vi "Write configuration.vi"(8 "error in":errorcluster, 10 "configuration":refnum<class "NISE_CEF_serializable configuration.lvclass">, 11 "My Awesome Control Modules editor node in":refnum<class "My Awesome Control Modules editor node.lvclass">) -> (0 "error out":errorcluster, 3 "My Awesome Control Modules editor node out":refnum<class "My Awesome Control Modules editor node.lvclass">)   [LabVIEW 2013, in "My Awesome Control Modules editor node.lvclass"]
uses:
  My Awesome Control Modules editor node.lvclass
  module/configuration/My Awesome Control Modules configuration.lvclass
  <vilib>/NI/Configuration Framework/serializable configuration/NISE_CEF_serializable configuration.lvclass
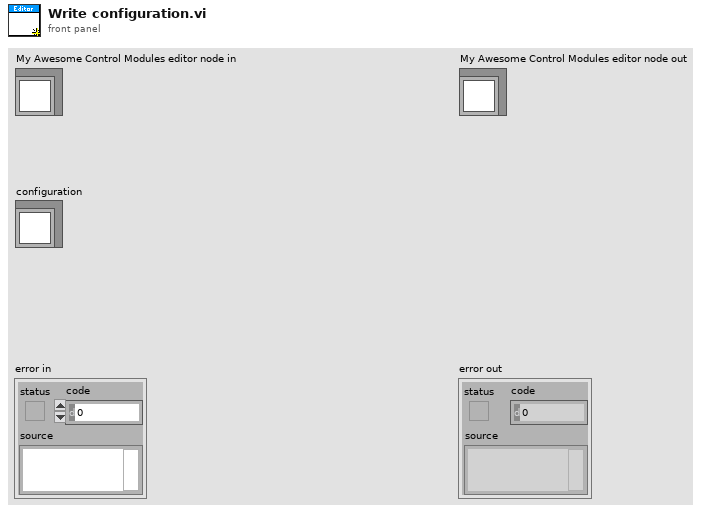
[diagram p1: front panel]
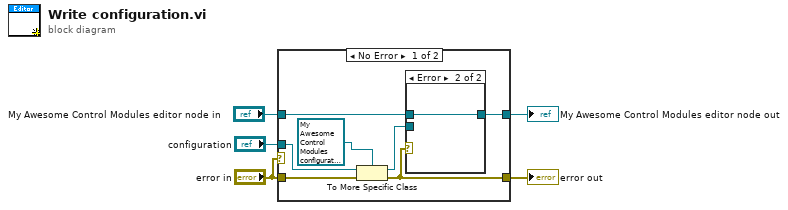
[diagram p0: block diagram]
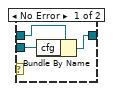
[diagram p2: hidden frame]
diagram:
  n1 = case shown="No Error" "error in" {
    tunnel: "error in" -> [w12 w18]
    tunnel: "My Awesome Control Modules editor node in" -> [w11 w17]
    tunnel: [w10 w17] -> w4
    tunnel: [w6 w18] -> w3
    tunnel: "configuration" -> [w9 _]
    frame No Error {
      n2 = To More Specific Class(target class=refnum<class "My Awesome Control Modules configuration.lvclass"> refnum ("module configuration"), reference=w9, error in=w12) -> (specific class reference=w7:refnum<class "My Awesome Control Modules configuration.lvclass">, error out=w6:errorcluster)
      n3 = case shown="Error" w6 {
        tunnel: w11 -> [w15 w16]
        tunnel: [w14 w16] -> w10
        tunnel: w7 -> [w13 _]
        frame No Error {
          n4 = Bundle By Name(cluster=w15, "cfg"=w13) -> (w14:refnum<class "My Awesome Control Modules editor node.lvclass">)
        }
        frame Error {
        }
      }
    }
    frame Error {
    }
  }
  "error out" <- w3
  "My Awesome Control Modules editor node out" <- w4
